vi "Parse Status Line.vi"(11 "Headers w/ status line":string) -> (0 "HTTP Version":string, 1 "HTTP Headers":string, 2 "Status String":string, 3 "Status Code":u16, 5 "Status Line":string)   [LabVIEW 2018, in "REST Client_JKI.lvlib" / "REST Client.lvclass"]
uses:
  REST Client.lvclass
  <vilib>/Utility/error.llb/whitespace.ctl
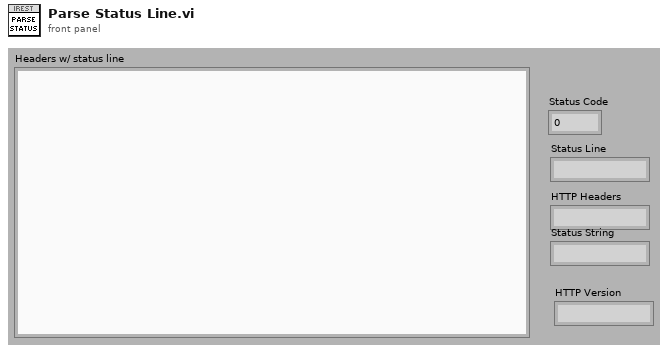
[diagram p1: front panel]
types:
  T1 = typedef "whitespace.ctl" = u16
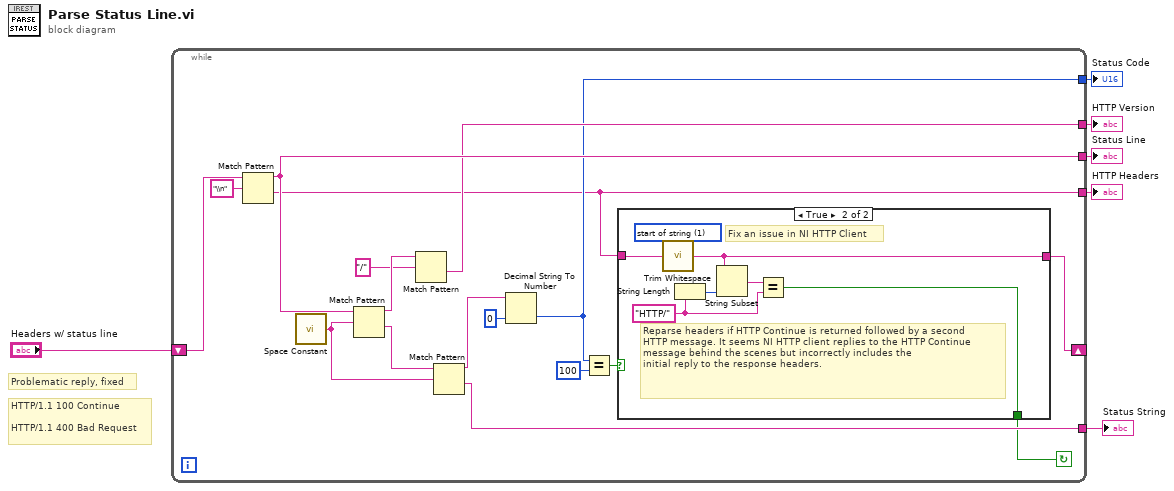
[diagram p0: block diagram]
diagram:
  # "Problematic reply, fixed"
  # "HTTP/1.1 100 Continue\n\nHTTP/1.1 400 Bad Request"
  n1 = while {
    shift-right: [w7] -> _
    shift-left: "Headers w/ status line" -> [w23]
    tunnel: [w22] -> w4
    tunnel: [w9] -> w5
    tunnel: [w19] -> w3
    tunnel: [w12] -> w1
    tunnel: [w16] -> w2
    stop <- w8 continue-if-true
    n2 = Match Pattern(string=w23, regular expression="\\n") -> (before substring=w22:string, after substring=w9:string)  [unwired: 1 in, 2 out]
    n3 = call <vilib>:"Space Constant.vi"() -> ("String"=w17:string)
    n4 = Match Pattern(string=w22, regular expression=w17) -> (before substring=w21:string, after substring=w18:string)  [unwired: 1 in, 2 out]
    n5 = Match Pattern(string=w21, regular expression="/") -> (after substring=w19:string)  [unwired: 1 in, 3 out]
    n6 = Match Pattern(string=w18, regular expression=w17) -> (before substring=w14:string, after substring=w16:string)  [unwired: 1 in, 2 out]
    n7 = Decimal String To Number(string=w14, default (0L)=u16 0 ("default (0 I32)")) -> (number=w12:u16)  [unwired: 1 in, 1 out]
    n8 = Equal?(x=w12, y=u16 100) -> (x = y?=w10:bool)
    n9 = case shown="True" w10 {
      tunnel: w9 -> [_ w29]
      tunnel: [_ w25] -> w8
      tunnel: [_ w24] -> w7
      frame False {
      }
      frame True {
        w26 = "HTTP/"
        w30 = T1 1 items=["both", "start of string", "end of string"] ("location (both)")
        # "Fix an issue in NI HTTP Client"
        # "Reparse headers if HTTP Continue is returned followed by a second\nHTTP message. It seems NI HTTP client replies to the HTTP Continue message behind the scenes but incorrectly includes the\ninitial reply to the response headers."
        n10 = call <vilib>:"Trim Whitespace.vi"("string"=w29, "location (both)"=w30) -> ("trimmed string"=w24:string)
        n11 = String Length(string=w26) -> (length=w28:i32)
        n12 = String Subset(string=w24, length (rest)=w28) -> (substring=w27:string)  [unwired: 1 in]
        n13 = Equal?(x=w27, y=w26) -> (x = y?=w25:bool)
      }
    }
  }
  "Status Line" <- w4
  "HTTP Headers" <- w5
  "HTTP Version" <- w3
  "Status String" <- w2
  "Status Code" <- w1
